vi "NumericOperations.vi"() -> ()   [LabVIEW 2019]
panel:
  out "Multiplication":dbl
  out "Subtraction":dbl
  out "Summation":dbl
  in  "number2":dbl
  in  "number1":dbl
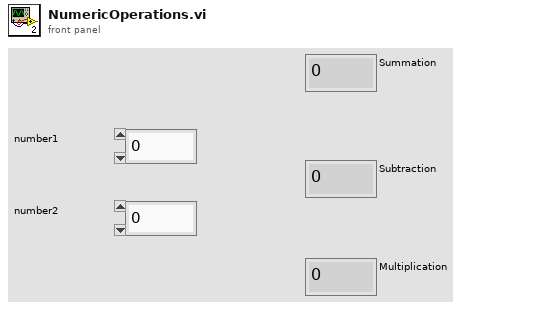
[diagram p1: front panel]
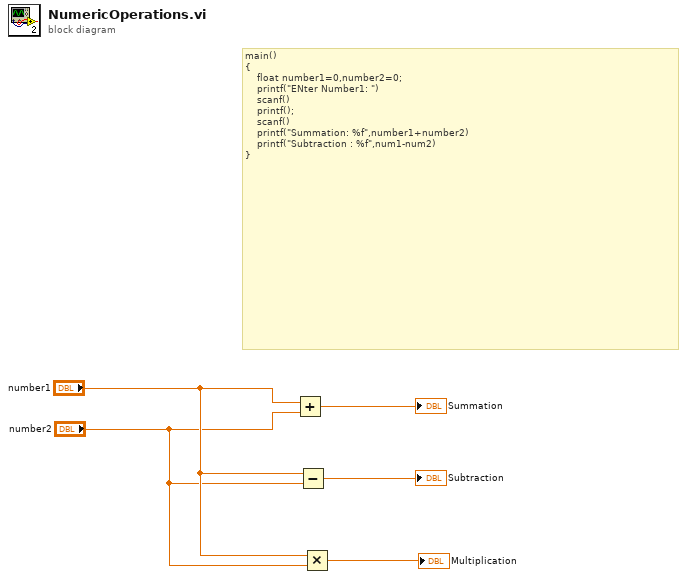
[diagram p0: block diagram]
diagram:
  # "main()\n{\n    float number1=0,number2=0;\n    printf(\"ENter Number1: \")\n    scanf()\n    printf();\n    scanf()\n    printf(\"Summation: %f\",number1+number2)\n    printf(\"Subtraction : %f\",num1-num2)\n}"
  n1 = Add(x="number1", y="number2") -> (x+y=→"Summation":dbl)
  n2 = Subtract(x="number1", y="number2") -> (x-y=→"Subtraction":dbl)
  n3 = Multiply(x="number1", y="number2") -> (x*y=→"Multiplication":dbl)
